vi "holding var.vi"() -> ()   [LabVIEW 2016, in "数据查询.lvlib"]
panel:
  in  "数据库备份位置":path=path "D:/sqlbackup"
  in  "自动备份":bool=TRUE
  in  "备份周期":enum16{"每小时", "每天", "每周", "每月"}(ring)
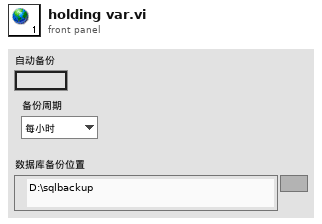
[diagram p1: front panel]
diagram:
